vi "closeRS232.vi"(1 "error in (no error)":errorcluster, 2 "VISA resource name":refnum<visa-resource-name>="COM1") -> ()   [LabVIEW 2011]
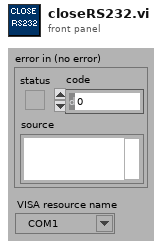
[diagram p1: front panel]
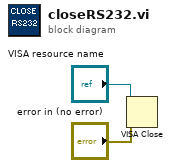
[diagram p0: block diagram]
diagram:
  n1 = VISA Close(VISA resource name="VISA resource name", error in (no error)="error in (no error)") -> ()  [unwired: 1 out]
